vi "MDrive Wait and Parse answer.vi"(8 "error in (no error)":errorcluster, 10 "Mdrive Mode":T1, 11 "VISA Refnum in":refnum<visa-resource-name>) -> (0 "error out":errorcluster, 2 "String":string, 3 "VISA Refnum out":refnum<visa-resource-name>)   [LabVIEW 2015]
uses:
  MDrive Mode.ctl
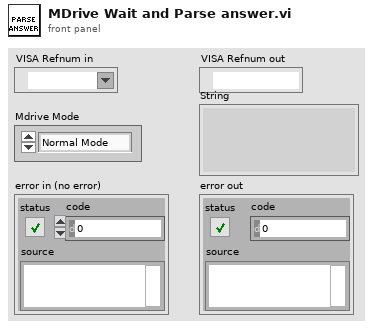
[diagram p1: front panel]
types:
  T1 = typedef "MDrive Mode.ctl" = enum16{"Normal Mode", "Party Mode"}
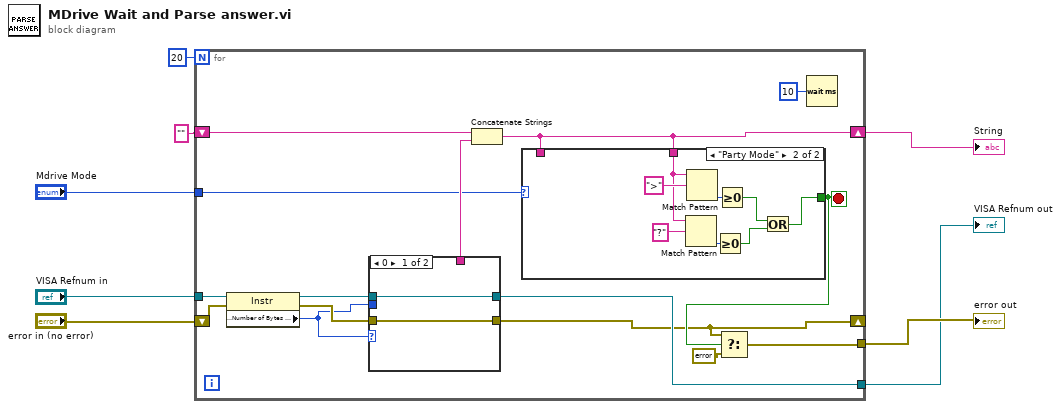
[diagram p0: block diagram]
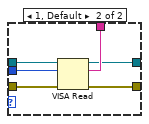
[diagram p2: hidden frame]
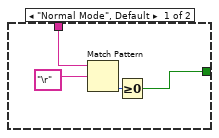
[diagram p3: hidden frame]
diagram:
  n1 = for {
    N: 20 -> [_]
    shift-right: [w9] -> w3
    shift-left: "" -> [w21]
    tunnel: "VISA Refnum in" -> [w23]
    tunnel: [w18] -> w4
    shift-right: [w13] -> _
    shift-left: "error in (no error)" -> [w16]
    tunnel: [w12] -> w7
    tunnel: "Mdrive Mode" -> [w11]
    stop <- w17 stop-if-true
    n2 = property class="Instr"(reference=w23, error in=w16) -> (reference out=w22:refnum<visa-resource-name>, error out=w15:errorcluster, "Serial Settings:Number of Bytes at Serial Port"=w10:u32)
    n3 = case shown="0" w10 {
      tunnel: w22 -> [w25 w31]
      tunnel: [_ w30] -> w20
      tunnel: [w25 w29] -> w18
      tunnel: w15 -> [w24 w28]
      tunnel: [w24 w27] -> w13
      tunnel: w10 -> [_ w26]
      frame 0 {
      }
      frame 1, Default {
        n4 = VISA Read(VISA resource name=w31, byte count=w26, error in (no error)=w28) -> (VISA resource name out=w29:refnum<visa-resource-name>, read buffer=w30:string, error out=w27:errorcluster)  [unwired: 1 out]
      }
    }
    n5 = Concatenate Strings(w21, w20) -> (w9:string)
    n6 = case shown="\"Party Mode\"" w11 {
      tunnel: w9 -> [w34 w36]
      tunnel: [w32 w37] -> w17
      tunnel: w9 -> [_ _]
      frame "Normal Mode", Default {
        n7 = Match Pattern(string=w34, regular expression="\r") -> (offset past match=w35:i32)  [unwired: 1 in, 3 out]
        n8 = Greater Or Equal To 0?(x=w35) -> (x >= 0?=w32:bool)
      }
      frame "Party Mode" {
        n9 = Match Pattern(string=w36, regular expression="?") -> (offset past match=w42:i32)  [unwired: 1 in, 3 out]
        n10 = Match Pattern(string=w36, regular expression=">") -> (offset past match=w43:i32)  [unwired: 1 in, 3 out]
        n11 = Greater Or Equal To 0?(x=w42) -> (x >= 0?=w38:bool)
        n12 = Greater Or Equal To 0?(x=w43) -> (x >= 0?=w39:bool)
        n13 = Or(x=w39, y=w38) -> (x .or. y?=w37:bool)
      }
    }
    n14 = Select(t=w13, s=w17, f=errorcluster {"status"=TRUE, "code"=0, "source"="Motor Failed"}) -> (s? t:f=w12:errorcluster)
    n15 = Wait (ms)(milliseconds to wait=u32 10) -> ()  [unwired: 1 out]
  }
  "error out" <- w7
  "VISA Refnum out" <- w4
  "String" <- w3
